vi "MC_Change_Selections.vi"(8 "error in (no error)":errorcluster, 9 "Point":T1, 11 "MCin":refnum<vi>) -> (0 "error out":errorcluster, 3 "MCout":refnum<vi>)   [LabVIEW 2013]
uses:
  <vilib>/Utility/miscctls.llb/LVPositionTypeDef.ctl
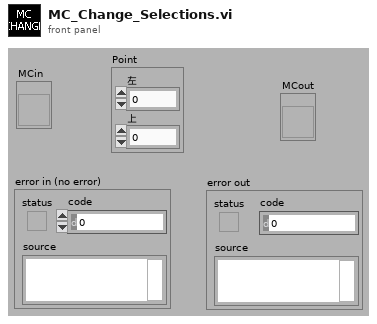
[diagram p1: front panel]
types:
  T1 = typedef "LVPositionTypeDef.ctl" = cluster{"Left":i32, "Top":i32}
  T2 = typedef "LVRowAndColumnTypeDef.ctl" = cluster{"Row":i32, "Column":i32}
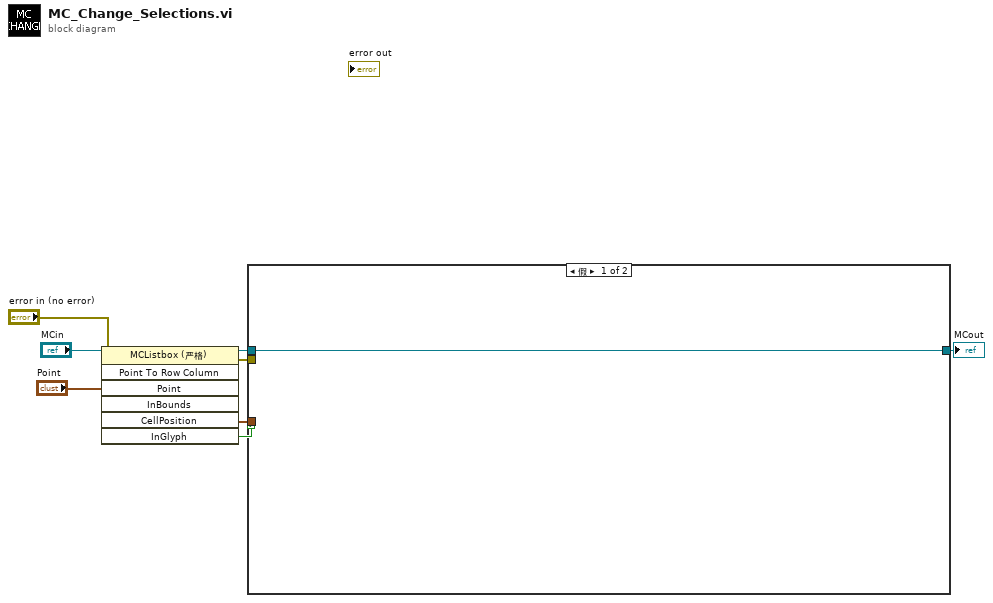
[diagram p0: block diagram]
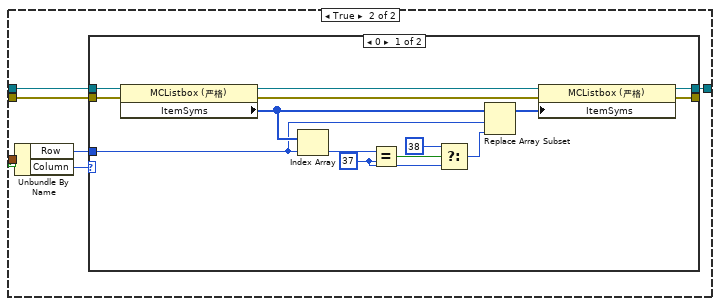
[diagram p2: hidden frame]
diagram:
  n1 = invoke on="调用节点" class="MCListbox (严格)" method="Point To Row Column"(reference="MCin", error in="error in (no error)", "Point"="Point") -> (reference out=w4:refnum<vi>, error out=w5:errorcluster, "CellPosition"=w8:T2, "InGlyph"=w1:bool)  [unwired: 4 in, 3 out]
  n2 = case shown="假" w1 {
    tunnel: w8 -> [_ w15]
    tunnel: w5 -> [_ w12]
    tunnel: w4 -> [w9 w11]
    tunnel: [w9 w10] -> w3
    frame False {
    }
    frame True {
      n3 = Unbundle By Name(w15) -> ("Row"=w13:i32, "Column"=w14:i32)
      n4 = case shown="0" w14 {
        tunnel: w13 -> [w23 _]
        tunnel: w12 -> [w21 w30]
        tunnel: w11 -> [w20 w31]
        tunnel: [w17 w30] -> _
        tunnel: [w16 w31] -> w10
        frame 0 {
          w28 = 37
          n5 = property on="属性节点" class="MCListbox (严格)"(reference=w20, error in=w21) -> (reference out=w19:refnum<vi>, error out=w18:errorcluster, "ItemSyms"=w25:i32[])
          n6 = Index Array(array=w25, index=w23) -> (element=w27:i32)
          n7 = Equal?(x=w27, y=w28) -> (x = y?=w29:bool)
          n8 = Select(t=38, s=w29, f=w28) -> (s? t:f=w24:i32)
          n9 = Replace Array Subset(array=w25, new element=w24, index=w23) -> (w22:i32[])
          n10 = property on="属性节点" class="MCListbox (严格)"(reference=w19, error in=w18, "ItemSyms"=w22) -> (reference out=w16:refnum<vi>, error out=w17:errorcluster)
        }
        frame 1, Default {
        }
      }
    }
  }
  "MCout" <- w3
